vi "update module id.vi"(8 "error in (no error)":errorcluster, 9 "New Id":string, 10 "Old Id":string, 11 "engine configuration in":refnum<class "engine configuration.lvclass">) -> (0 "error out":errorcluster, 3 "engine configuration out":refnum<class "engine configuration.lvclass">)   [LabVIEW 2013, in "engine configuration.lvclass"]
uses:
  engine configuration.lvclass
  engine configuration.lvclass/engine configuration.ctl
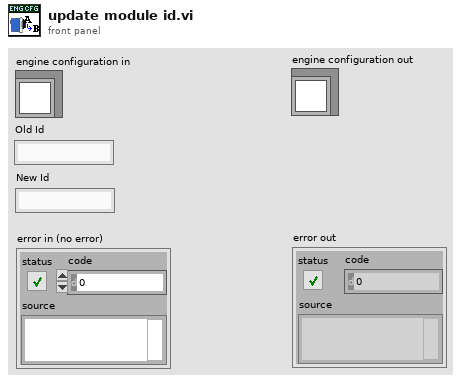
[diagram p1: front panel]
types:
  T1 = typedef "engine configuration.lvclass/module channel pairings.ctl" = cluster{"modules":string[], "channels":string[]}
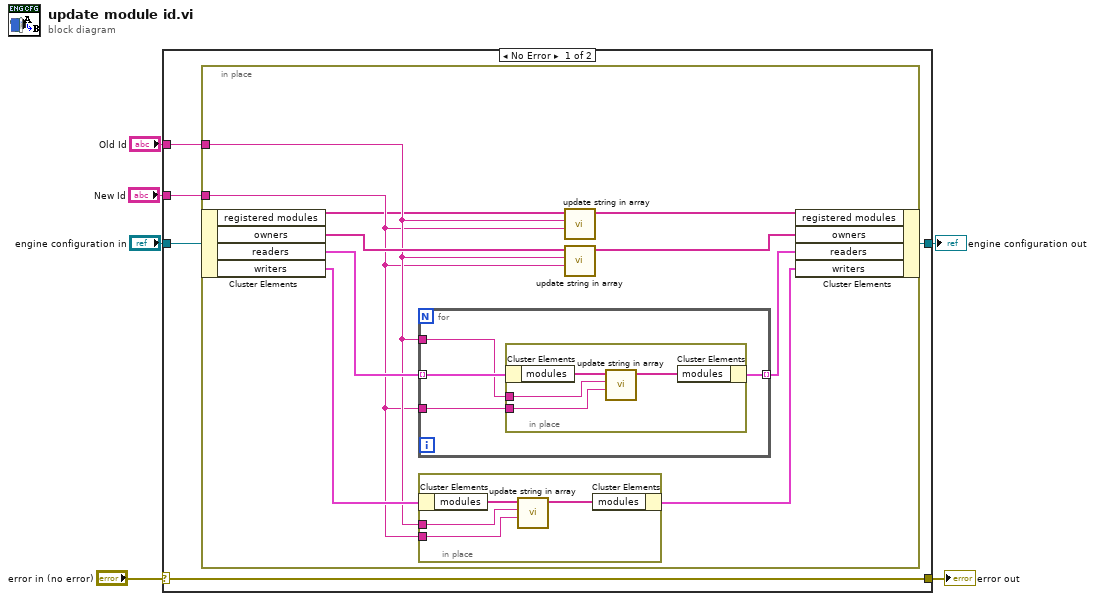
[diagram p0: block diagram]
diagram:
  n1 = case shown="No Error" "error in (no error)" {
    selector: "error in (no error)" -> [w7 w35]
    tunnel: "engine configuration in" -> [w11 w34]
    tunnel: "Old Id" -> [w10 _]
    tunnel: "New Id" -> [w9 _]
    tunnel: [w8 w34] -> w3
    tunnel: [w7 w35] -> w1
    frame No Error {
      n2 = in-place {
        in-place-border: w10 -> [w16]
        in-place-border: w9 -> [w15]
        n3 = in-place-cluster #1(w11) -> ("registered modules"=w14:string[], "owners"=w18:string[], "readers"=w19:T1[], "writers"=w21:T1)
        n4 = for {
          tunnel: w19 -> [w25] mode=indexing
          tunnel: [w24] -> w12 mode=indexing
          tunnel: w16 -> [w23]
          tunnel: w15 -> [w22]
          n5 = in-place {
            in-place-border: w23 -> [w27]
            in-place-border: w22 -> [w26]
            n6 = in-place-cluster #2(w25) -> ("modules"=w29:string[])
            n7 = call "update string in array.vi"("New Id"=w26, "Old Id"=w27, "registered modules"=w29) -> ("Array"=w28:string[])  [unwired: 8 in]
            n8 = in-place-cluster #2("modules"=w28) -> (w24:T1)
          }
        }
        n9 = in-place {
          in-place-border: w16 -> [w31]
          in-place-border: w15 -> [w30]
          n10 = in-place-cluster #3(w21) -> ("modules"=w33:string[])
          n11 = call "update string in array.vi"("New Id"=w30, "Old Id"=w31, "registered modules"=w33) -> ("Array"=w32:string[])  [unwired: 8 in]
          n12 = in-place-cluster #3("modules"=w32) -> (w20:T1)
        }
        n13 = call "update string in array.vi"("New Id"=w15, "Old Id"=w16, "registered modules"=w14) -> ("Array"=w13:string[])  [unwired: 8 in]
        n14 = call "update string in array.vi"("New Id"=w15, "Old Id"=w16, "registered modules"=w18) -> ("Array"=w17:string[])  [unwired: 8 in]
        n15 = in-place-cluster #1("registered modules"=w13, "owners"=w17, "readers"=w12, "writers"=w20) -> (w8:refnum<class "engine configuration.lvclass">)
      }
    }
    frame Error {
    }
  }
  "engine configuration out" <- w3
  "error out" <- w1
